vi "SwapIntoArray.vi"(8 "element in":T1, 9 "index":i32, 11 "PipeData in":refnum<class "StreamData.lvclass">) -> (0 "element out":T1, 3 "PipeData out":refnum<class "StreamData.lvclass">)   [LabVIEW 2017, in "Stream-t'WPI_EncoderType.ctl'.lvlib" / "StreamData.lvclass"]
uses:
  <extravilib>/ChannelInstances/Stream-t'WPI_EncoderType.ctl'/StreamData.lvclass
  <vilib>/Rock Robotics/WPI/Encoder/WPI_EncoderType.ctl
  <extravilib>/ChannelInstances/Stream-t'WPI_EncoderType.ctl'/StreamData.lvclass/StreamData.ctl
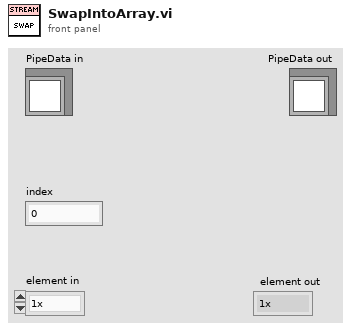
[diagram p1: front panel]
types:
  T1 = typedef "WPI_EncoderType.ctl" = enum16{"1x", "2x", "4x"}
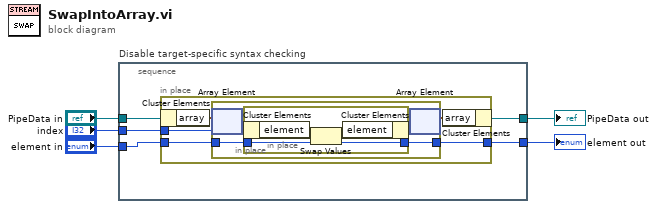
[diagram p0: block diagram]
diagram:
  n1 = stacked-sequence "Disable target-specific syntax checking" {
    tunnel: [w10] -> w5
    tunnel: "PipeData in" -> [w9]
    tunnel: "index" -> [w8]
    tunnel: "element in" -> [w7]
    tunnel: [w6] -> w1
    frame #0 {
      n2 = in-place {
        in-place-border: [w14] -> w6
        in-place-border: w7 -> [w13]
        in-place-border: w8 -> [w11]
        n3 = in-place-cluster #1(w9) -> ("array"=w12:cluster{"element":T1}[])
        n4 = in-place {
          in-place-border: w13 -> [w19]
          in-place-border: [w18] -> w14
          n5 = in-place-array #2(w12, w11) -> (w17:cluster{"element":T1})
          n6 = in-place {
            in-place-border: w19 -> [w23]
            in-place-border: [w22] -> w18
            n7 = in-place-cluster #3(w17) -> ("element"=w21:T1)
            n8 = Swap Values(12:w21, 14:w23) -> (1:w20:T1, 3:w22:T1)  [unwired: 1 in]
            n9 = in-place-cluster #3("element"=w20) -> (w16:cluster{"element":T1})
          }
          n10 = in-place-array #2(w16) -> (w15:cluster{"element":T1}[])  [unwired: 1 out]
        }
        n11 = in-place-cluster #1("array"=w15) -> (w10:refnum<class "StreamData.lvclass">)
      }
    }
  }
  "PipeData out" <- w5
  "element out" <- w1
